vi "grabber.vi"() -> ()   [LabVIEW 2010]
uses:
  status_enum.ctl
  type definitions/command_enum.ctl
  <vilib>/rvi/interface/nirviReadWriteControl/nirviReadWriteControl.xnode
  FPGA_VI_reference.ctl
  <vilib>/rvi/interface/common/niFpgaNodeNameForErrorReporting.ctl
  <vilib>/rvi/errors/niLvFpgaWhatHappensToTopLevelVI.ctl
  <vilib>/dex/Flush And Wait Empty Condition.ctl
  <vilib>/rvi/interface/nirviMethod/nirviMethod.xnode
  <vilib>/rvi/interface/nirviCloseFPGA/nirviCloseFPGA.xnode
  <vilib>/Utility/error.llb/Error Cluster From Error Code.vi
  <vilib>/rvi/errors/niLvFpgaAdjustHostInterfaceError.vi
  <vilib>/FPGAPlugInAG/Dynamic/niLvFpga_Close_Dynamic.vi
  NiFpgaLv.dll
panel:
  out "channel 3":u32
  out "channel 2":u32
  out "channel 1":u32
  out "channel 0":u32
  out "triggered flag valid?":bool
  out "triggered?":bool
  out "pixel frequency (Hz)":dbl
  out "number of pixels":i64
  out "loop counter":i32
  in  "writer buffer size":i32=1000000 format="%.0e"
  in  "Close front-panel?":bool=TRUE
  out "pixel counter":i64
  out "data read":u64[](array[numeric])
  out "last command during acquisition":T1
  out "last command":T1
  out "state":T2
  out "FIFO overflow":bool
  out "error out":errorcluster
  # "Grabber.exe of FPGAWrapperDL120115Galvo\n\n\nAuthor: Dominik Langer\ncopyright: University of Zurich, Switzerland"
  # "Grabber.exe"
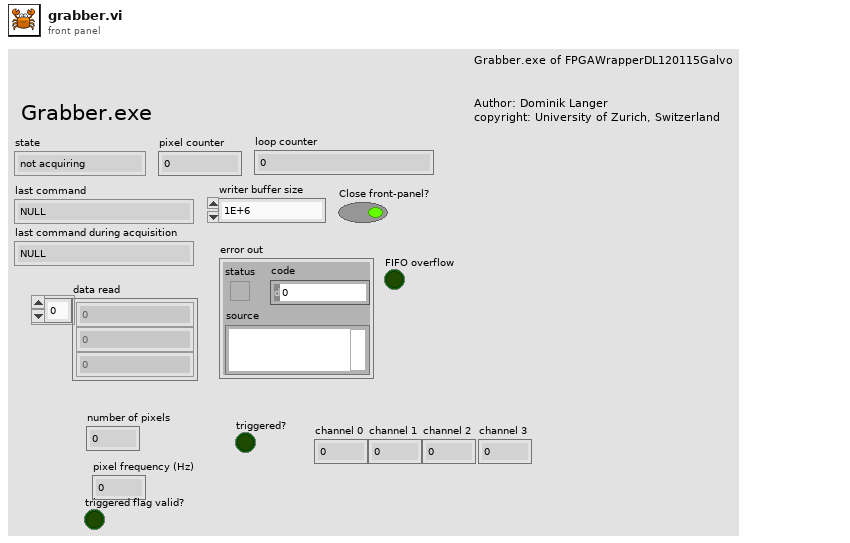
[diagram p1: front panel]
types:
  T1 = typedef "command_enum.ctl" = enum16{"NULL", "update", "start", "stop", "reset", "shut-down"}
  T2 = typedef "status_enum.ctl" = enum16{"not acquiring", "acquiring"}
  T3 = typedef "network_streaming_queues_cluster.ctl" = cluster{"configuration reader endpoint":refnum<k21>, "settings reader endpoint":refnum<k21>, "data writer endpoint":refnum<k21>, "command reader endpoint":refnum<k21>}
  T4 = typedef "FPGA_VI_reference.ctl" = refnum<k20>
  T5 = typedef "niFpgaNodeNameForErrorReporting.ctl" = enum16{"Open FPGA VI Reference", "Read/Write Control", "Invoke Method: Abort", "Invoke Method: Acknowledge IRQ", "Invoke Method: Download", "Invoke Method: FIFO.Configure", "Invoke Method: FIFO.Read", "Invoke Method: FIFO.Start", "Invoke Method: FIFO.Stop", "Invoke Method: FIFO.Write", "Invoke Method: Reset", "Invoke Method: Run", "Invoke Method: Wait on IRQ", "Close FPGA VI Reference"}
  T6 = typedef "niLvFpgaWhatHappensToTopLevelVI.ctl" = enum16{"top level VI scripted behind XNode", "top level VI inlined behind XNode"}
  T7 = typedef "settings_cluster.ctl" = cluster{"number of pixels":i64, "pixel frequency (Hz)":dbl, "pixel values cluster":T8, "triggered?":bool, "triggered flag valid?":bool, "gates":T9[]}
  T8 = typedef "channels_cluster.ctl" = cluster{"channel 0":u32, "channel 1":u32, "channel 2":u32, "channel 3":u32}
  T9 = typedef "gate_cluster.ctl" = cluster{"index":i32, "parameters":T10}
  T10 = typedef "gate_parameters_cluster.ctl" = cluster{"offset":i64, "pulsing":i64, "not pulsing":i64, "cycles per pulse":i64, "repetitions":i64}
  T11 = typedef "Flush And Wait Empty Condition.ctl" = u8
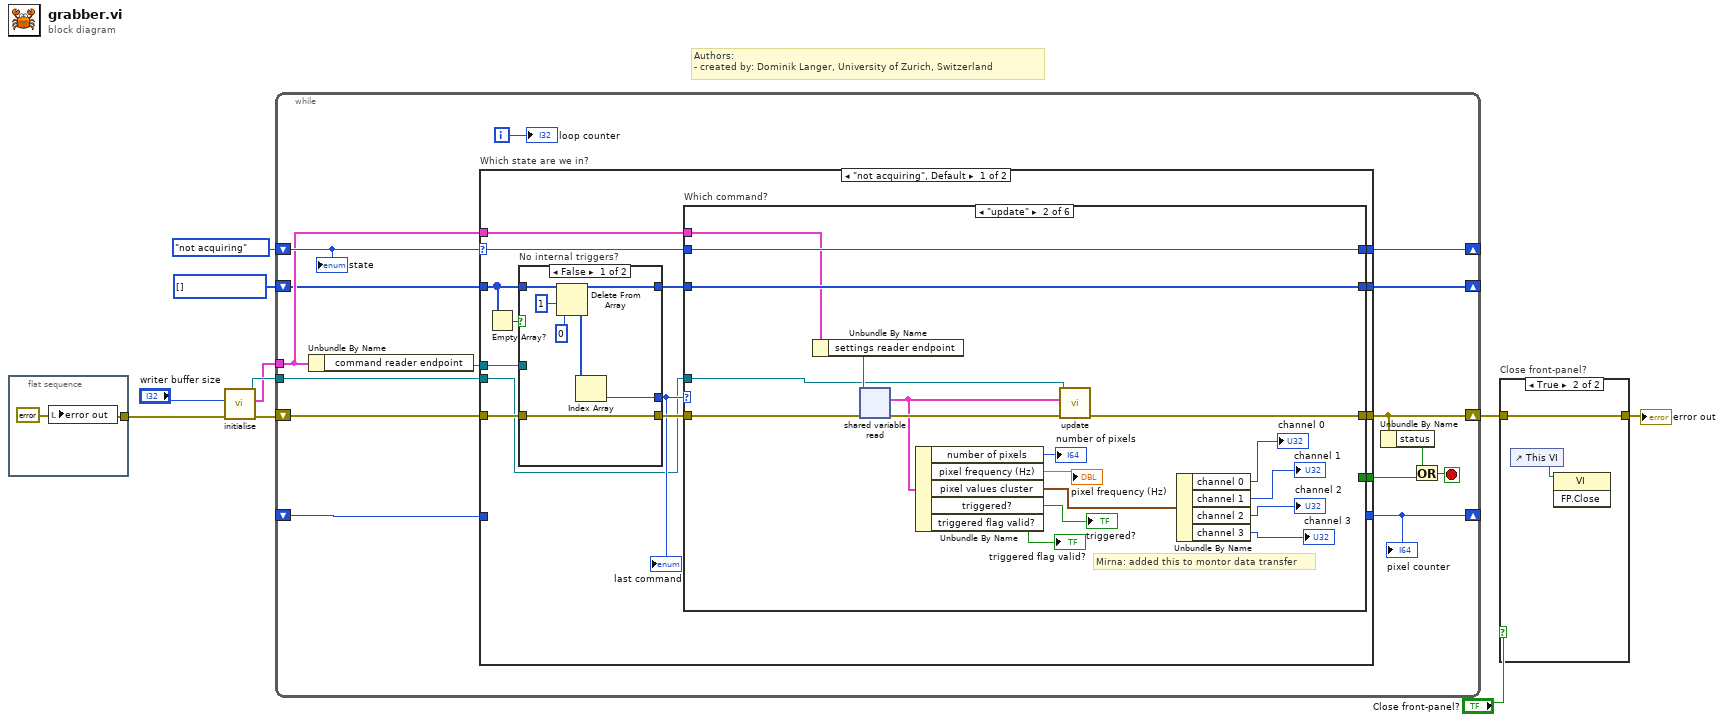
[diagram p0: block diagram]
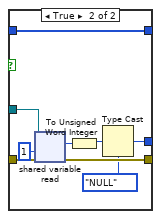
[diagram p2: hidden frame]
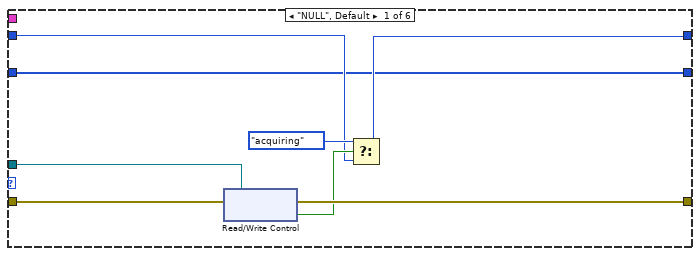
[diagram p3: hidden frame]
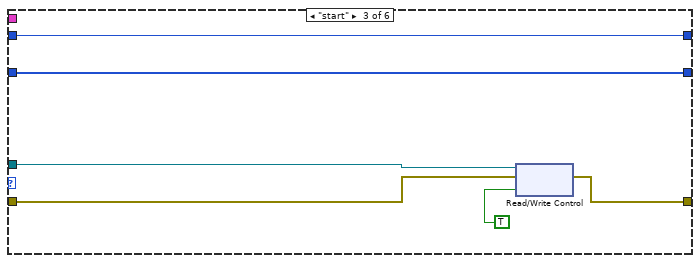
[diagram p4: hidden frame]
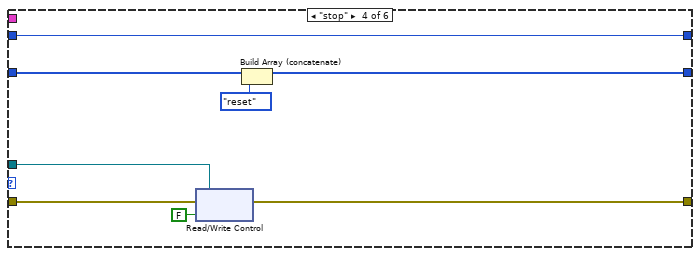
[diagram p5: hidden frame]
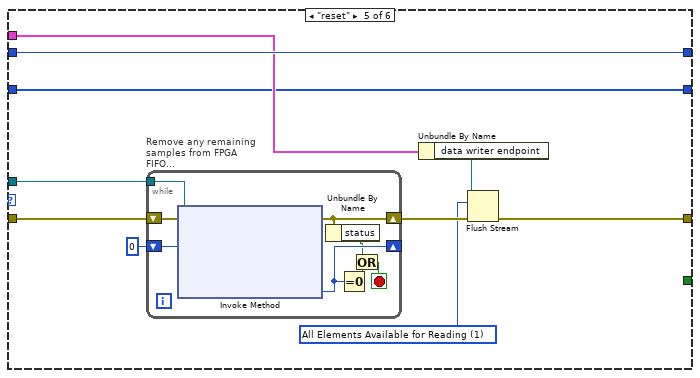
[diagram p6: hidden frame]
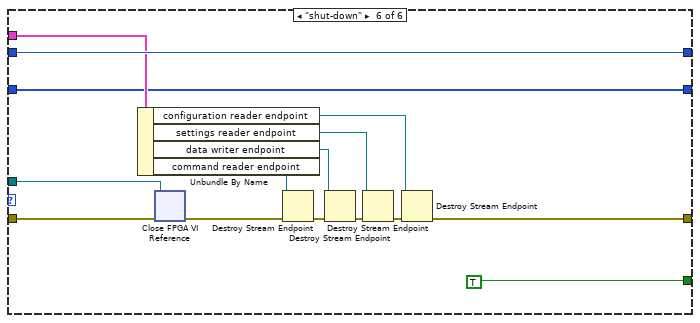
[diagram p7: hidden frame]
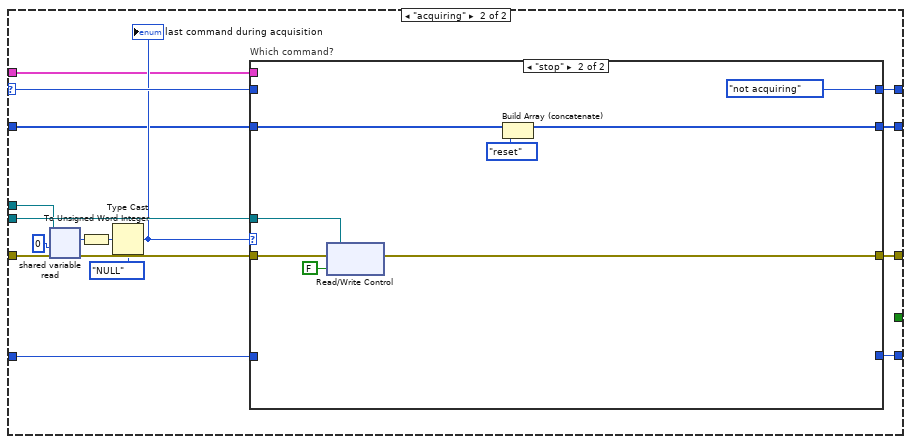
[diagram p8: hidden frame]
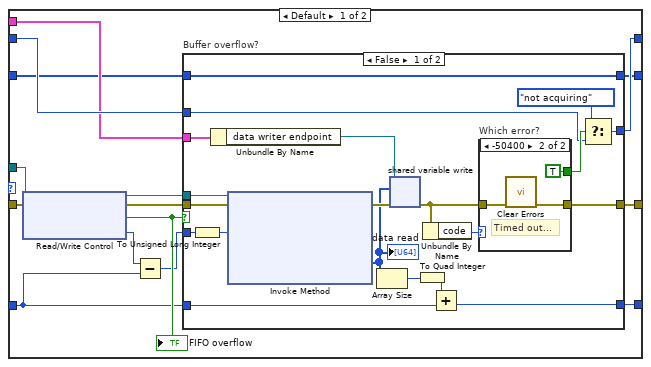
[diagram p9: hidden frame]
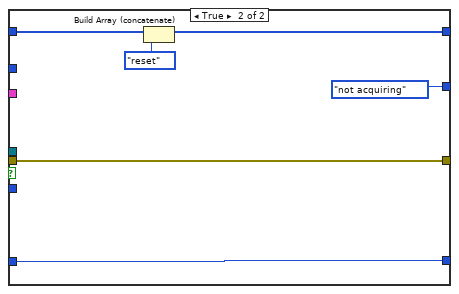
[diagram p11: hidden frame]
diagram:
  w1 = T1[] [] items=["NULL", "update", "start", "stop", "reset", "shut-down"]
  # "Authors: \n- created by: Dominik Langer, University of Zurich, Switzerland"
  n1 = flat-sequence {
    tunnel: [w11] -> w6
    frame #0 {
      w11 = errorcluster {"status"=FALSE, "code"=0, "source"=""} ("error in (no error)")
      n2 = local write "error out"(w11) -> ()
    }
  }
  n3 = call "initialise.vi"("error in (no error)"=w6, "writer buffer size"="writer buffer size") -> ("error out"=w5:errorcluster, "network streaming queues"=w2:T3, "FPGA VI Reference Out"=w3:T4)  [unwired: 7 in]
  n4 = while {
    shift-right: [w22] -> w7
    shift-left: w5 -> [w14]
    shift-right: [w24] -> _
    shift-left: status_enum."not acquiring" ("status") -> [w26]
    tunnel: w3 -> [w25]
    shift-right: [w18] -> _
    shift-left: _ -> [w23]
    tunnel: w2 -> [w16]
    shift-right: [w13] -> _
    shift-left: w1 -> [w12]
    i -> [w17]
    stop <- w19 stop-if-true
    n5 = Unbundle By Name(w16) -> ("command reader endpoint"=w15:refnum<k21>)
    n6 = case "Which state are we in?" shown="\"not acquiring\", Default" w26 {
      selector: w26 -> [w36 w344]
      tunnel: w14 -> [w39 w342]
      tunnel: [w40 w345] -> w22
      tunnel: w25 -> [w34 w346]
      tunnel: w15 -> [w31 w340]
      tunnel: [w35 w343] -> w24
      tunnel: w23 -> [_ w335]
      tunnel: [w33 _] -> w21
      tunnel: [_ w334] -> w18
      tunnel: w16 -> [w32 w333]
      tunnel: [w30 w331] -> w13
      tunnel: w12 -> [w28 w330]
      frame "not acquiring", Default {
        n7 = Empty Array?(array=w28) -> (empty?=w27:bool)
        n8 = case "No internal triggers?" shown="False" w27 {
          tunnel: w39 -> [w47 w54]
          tunnel: [w47 w53] -> w38
          tunnel: [w42 w52] -> w37
          tunnel: w31 -> [_ w51]
          tunnel: w28 -> [w46 w48]
          tunnel: [w41 w48] -> w29
          frame False {
            n9 = Delete From Array(array=w46, length=1, index=0) -> (deleted portion=w43:T1[], array with subset deleted=w41:T1[])
            n10 = Index Array(array=w43) -> (element=w42:T1)  [unwired: 1 in]
          }
          frame True {
            n11 = shared-variable-read(w51, w54, 1 ("timeout in ms (-1)")) -> (w53:errorcluster, w55:u32)  [unwired: 2 out]
            n12 = To Unsigned Word Integer(number=w55) -> (unsigned 16bit integer=w56:u16)
            n13 = Type Cast(type=command_enum."NULL" ("command"), x=w56) -> (*(type *) &x=w52:T1)
          }
        }
        "last command" <- w37
        n14 = case "Which command?" shown="\"update\"" w37 {
          tunnel: w38 -> [w64 w124 w126 w176 w224 w320]
          tunnel: [w63 w122 w130 w175 w221 w317] -> w40
          tunnel: w36 -> [w60 w125 w129 w178 w227 w323]
          tunnel: [w59 w125 w129 w178 w227 w323] -> w35
          tunnel: w34 -> [w58 w108 w127 w174 w226 w321]
          tunnel: [_ _ _ _ _ TRUE] -> w33
          tunnel: w32 -> [_ w119 _ _ w220 w314]
          tunnel: w29 -> [w57 w120 w128 w173 w218 w309]
          tunnel: [w57 w120 w128 w171 w218 w309] -> w30
          frame "NULL", Default {
            n15 = xnode "Read/Write Control"("FPGA VI Reference In"=w58, "error in"=w64) -> ("error out"=w63:errorcluster, "acquiring?"=w62:bool)  [unwired: 1 out]
            n16 = Select(t=status_enum."acquiring" ("status"), s=w62, f=w60) -> (s? t:f=w59:T2)
          }
          frame "update" {
            # "Mirna: added this to montor data transfer"
            n17 = Unbundle By Name(w119) -> ("settings reader endpoint"=w121:refnum<k21>)
            n18 = shared-variable-read(w121, w124) -> (w123:errorcluster, w118:T7)  [unwired: 1 in, 2 out]
            n19 = Unbundle By Name(w118) -> ("number of pixels"=→"number of pixels":i64, "pixel frequency (Hz)"=→"pixel frequency (Hz)":dbl, "pixel values cluster"=w113:T8, "triggered?"=→"triggered?":bool, "triggered flag valid?"=→"triggered flag valid?":bool)
            n20 = call "update.vi"("error in"=w123, "settings cluster"=w118, "FPGA VI ref"=w108) -> ("error out"=w122:errorcluster)  [unwired: 8 in]
            n21 = Unbundle By Name(w113) -> ("channel 0"=→"channel 0":u32, "channel 1"=→"channel 1":u32, "channel 2"=→"channel 2":u32, "channel 3"=→"channel 3":u32)
          }
          frame "start" {
            n22 = xnode "Read/Write Control"("FPGA VI Reference In"=w127, "error in"=w126, "acquire"=TRUE) -> ("error out"=w130:errorcluster)  [unwired: 1 out]
          }
          frame "stop" {
            n23 = xnode "Read/Write Control"("FPGA VI Reference In"=w174, "error in"=w176, "acquire"=FALSE) -> ("error out"=w175:errorcluster)  [unwired: 1 out]
            n24 = Build Array (concatenate)(w173, command_enum."reset" ("command")) -> (w171:T1[])
          }
          frame "reset" {
            w219 = T11 1 items=["All Elements Read From Stream", "All Elements Available for Reading"] ("wait condition")
            n25 = while "Remove any remaining samples from FPGA FIFO..." {
              tunnel: w226 -> [w234]
              shift-right: [w232] -> _
              shift-left: u32 0 ("Elements Remaining") -> [w233]
              shift-right: [w231] -> w222
              shift-left: w224 -> [w235]
              stop <- w228 stop-if-true
              n26 = xnode "Invoke Method"("FPGA VI Reference In"=w234, "error in"=w235, "Number of Elements"=w233) -> ("error out"=w231:errorcluster, "Elements Remaining"=w232:u32)  [unwired: 1 in, 2 out]
              n27 = Unbundle By Name(w231) -> ("status"=w229:bool)
              n28 = Equal To 0?(x=w232) -> (x = 0?=w230:bool)
              n29 = Or(x=w229, y=w230) -> (x .or. y?=w228:bool)
            }
            n30 = Unbundle By Name(w220) -> ("data writer endpoint"=w223:refnum<k21>)
            n31 = Flush Stream(8:w222, 10:w219, 11:w223) -> (0:w221:errorcluster)  [unwired: 1 in, 2 out]
          }
          frame "shut-down" {
            n32 = Unbundle By Name(w314) -> ("configuration reader endpoint"=w310:refnum<k21>, "settings reader endpoint"=w311:refnum<k21>, "data writer endpoint"=w312:refnum<k21>, "command reader endpoint"=w313:refnum<k21>)
            n33 = xnode "Close FPGA VI Reference"("FPGA VI Reference In"=w321, "error in"=w320) -> ("error out"=w319:errorcluster)
            n34 = Destroy Stream Endpoint(8:w319, 11:w313) -> (0:w318:errorcluster)
            n35 = Destroy Stream Endpoint(8:w318, 11:w312) -> (0:w316:errorcluster)
            n36 = Destroy Stream Endpoint(8:w316, 11:w311) -> (0:w315:errorcluster)
            n37 = Destroy Stream Endpoint(8:w315, 11:w310) -> (0:w317:errorcluster)
          }
        }
      }
      frame "acquiring" {
        n38 = shared-variable-read(w340, w342, 0 ("timeout in ms (-1)")) -> (w341:errorcluster, w339:u32)  [unwired: 2 out]
        n39 = To Unsigned Word Integer(number=w339) -> (unsigned 16bit integer=w338:u16)
        n40 = Type Cast(type=command_enum."NULL" ("command"), x=w338) -> (*(type *) &x=w336:T1)
        "last command during acquisition" <- w336
        n41 = case "Which command?" shown="\"stop\"" w336 {
          tunnel: w346 -> [w359 w544]
          tunnel: [w358 w545] -> w345
          tunnel: w344 -> [w357 _]
          tunnel: [w356 status_enum."not acquiring" ("status")] -> w343
          tunnel: w341 -> [w355 w546]
          tunnel: w335 -> [w349 _]
          tunnel: [w353 _] -> w334
          tunnel: w333 -> [w350 _]
          tunnel: [w347 w541] -> w331
          tunnel: w330 -> [w348 w543]
          frame Default {
            n42 = xnode "Read/Write Control"("FPGA VI Reference In"=w359, "error in"=w355) -> ("FPGA VI Reference Out"=w360:T4, "error out"=w361:errorcluster, "FIFO overflow"=w354:bool, "current pixel no."=w352:i64)
            "FIFO overflow" <- w354
            n43 = Subtract(x=w352, y=w349) -> (x-y=w351:i64)
            n44 = case "Buffer overflow?" shown="False" w354 {
              tunnel: w361 -> [w381 w464]
              tunnel: w360 -> [w380 _]
              tunnel: [w378 w464] -> w358
              tunnel: w357 -> [w366 _]
              tunnel: [w364 status_enum."not acquiring" ("status")] -> w356
              tunnel: w349 -> [w374 w462]
              tunnel: [w373 w462] -> w353
              tunnel: w351 -> [w371 _]
              tunnel: w350 -> [w369 _]
              tunnel: w348 -> [w362 w461]
              tunnel: [w362 w459] -> w347
              frame False {
                n45 = To Unsigned Long Integer(number=w371) -> (unsigned 32bit integer=w370:u32)
                n46 = Unbundle By Name(w369) -> ("data writer endpoint"=w368:refnum<k21>)
                n47 = xnode "Invoke Method"("FPGA VI Reference In"=w380, "error in"=w381, "Number of Elements"=w370) -> ("error out"=w377:errorcluster, "Data"=w363:u64[])  [unwired: 1 in, 2 out]
                "data read" <- w363
                n48 = Array Size(array=w363) -> (size(s)=w375:i32)
                n49 = shared-variable-write(w368, w377, w363) -> (w376:errorcluster)  [unwired: 1 in, 2 out]
                n50 = To Quad Integer(1:w375) -> (0:w372:i64)
                n51 = Unbundle By Name(w376) -> ("code"=w379:i32)
                n52 = Add(x=w372, y=w374) -> (x+y=w373:i64)
                n53 = case "Which error?" shown="-50400" w379 {
                  tunnel: [w382 w384] -> w378
                  tunnel: w376 -> [w382 w385]
                  tunnel: [_ TRUE] -> w367
                  frame 0, Default {
                  }
                  frame -50400 {
                    # "Timed out..."
                    n54 = call <vilib>:"Clear Errors.vi"("error in (no error)"=w385) -> ("error out"=w384:errorcluster)  [unwired: 6 in]
                  }
                }
                n55 = Select(t=status_enum."not acquiring" ("status"), s=w367, f=w366) -> (s? t:f=w364:T2)
              }
              frame True {
                n56 = Build Array (concatenate)(w461, command_enum."reset" ("command")) -> (w459:T1[])
              }
            }
          }
          frame "stop" {
            n57 = xnode "Read/Write Control"("FPGA VI Reference In"=w544, "error in"=w546, "acquire"=FALSE) -> ("error out"=w545:errorcluster)  [unwired: 1 out]
            n58 = Build Array (concatenate)(w543, command_enum."reset" ("command")) -> (w541:T1[])
          }
        }
      }
    }
    "pixel counter" <- w18
    n59 = Unbundle By Name(w22) -> ("status"=w20:bool)
    n60 = Or(x=w20, y=w21) -> (x .or. y?=w19:bool)
    "state" <- w26
    "loop counter" <- w17
  }
  n61 = case "Close front-panel?" shown="True" "Close front-panel?" {
    tunnel: [w588 w589] -> w8
    tunnel: w7 -> [w588 w589]
    frame False {
    }
    frame True {
      n62 = control-ref of="This VI"() -> (w590:refnum<vi>)
      n63 = invoke class="VI" method="FP.Close"(reference=w590) -> ()  [unwired: 2 in, 3 out]
    }
  }
  "error out" <- w8
